vi "Start Batch Process.vi"(8 "error in (no error)":errorcluster, 10 "Files to process":path[](array[path]), 11 "Batch Processor in":refnum<class "Batch Processor.lvclass">) -> (0 "error out":errorcluster, 3 "Batch Processor out":refnum<class "Batch Processor.lvclass">)   [LabVIEW 2016, in "Batch Processor.lvclass"]
uses:
  Batch Processor.lvclass
  C:/Github/LabActor/Worker/Worker.lvclass
  NHMFL_Core/Libraries/Instruments/Instrument Driver/Worker State.ctl
  Worker/Worker.lvclass/Worker.ctl
  NHMFL_Core/Libraries/Instruments/Results/File Path Result/File Path Result.lvclass
  C:/Github/NHMFL_Core/Libraries/Instruments/Results/Acquired Result/Acquired Result.lvclass
  Batch Processor.lvclass/Batch Processor.ctl
  Template Module/Read State.vi
  Template Module/Write State.vi
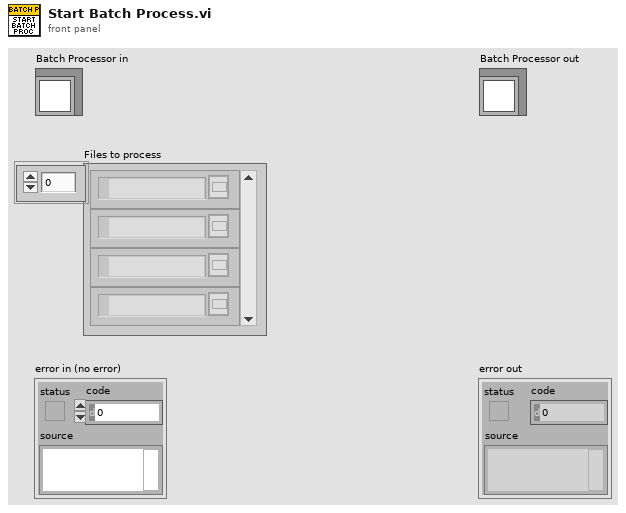
[diagram p1: front panel]
types:
  T1 = typedef "Worker State.ctl" = enum16{"Idle", "Starting", "Working", "Stopping"}
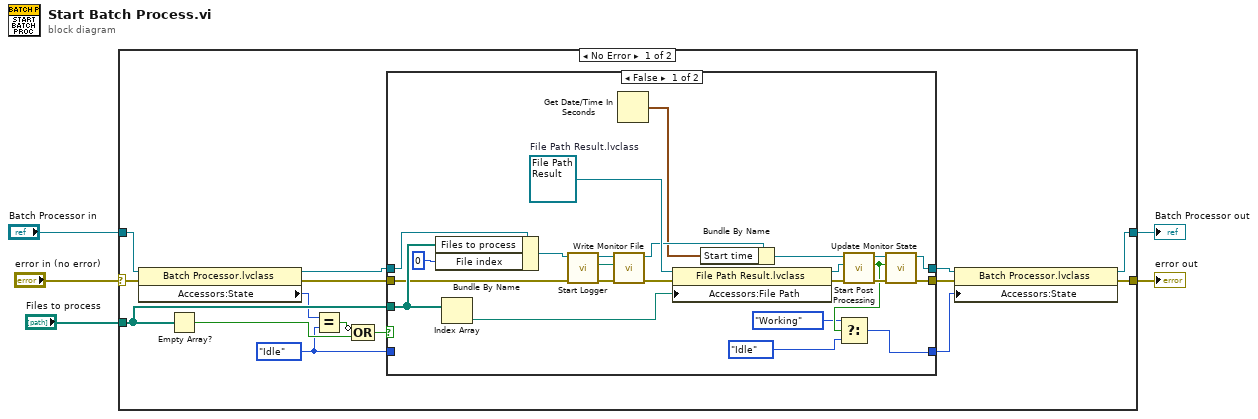
[diagram p0: block diagram]
diagram:
  n1 = case shown="No Error" "error in (no error)" {
    selector: "error in (no error)" -> [w20 w49]
    tunnel: [w6 w49] -> w4
    tunnel: [w7 w48] -> w2
    tunnel: "Batch Processor in" -> [w16 w48]
    tunnel: "Files to process" -> [w19 _]
    frame No Error {
      w9 = Worker_State."Idle" ("State")
      n2 = property class="Batch Processor.lvclass"(reference=w16, error in=w20) -> (reference out=w15:refnum<class "Batch Processor.lvclass">, error out=w17:errorcluster, "Accessors:State"=w12:T1)
      n3 = Empty Array?(array=w19) -> (empty?=w18:bool)
      n4 = Equal?(x=w12, y=w9) -> (x = y?=w13:bool)
      n5 = Compound Arithmetic op=OR(invert w13, w18) -> (w14:bool)
      n6 = case shown="False" w14 {
        tunnel: w15 -> [w44 w46]
        tunnel: w19 -> [w41 _]
        tunnel: w17 -> [w36 w47]
        tunnel: [w29 w46] -> w11
        tunnel: [w28 w47] -> w8
        tunnel: [w23 w45] -> w10
        tunnel: w9 -> [_ w45]
        frame False {
          w42 = refnum<class "File Path Result.lvclass"> refnum  # File Path Result.lvclass
          n7 = Bundle By Name(cluster=w44, "Files to process"=w41, "File index"=0) -> (w37:refnum<class "Batch Processor.lvclass">)
          n8 = Index Array(array=w41) -> (element=w40:path)  [unwired: 1 in]
          n9 = call-dynamic "Start Logger.vi"("error in (no error)"=w36, "Measure Controller in"=w37) -> ("error out"=w33:errorcluster, "File Path"=w31:path, "Measure Controller out"=w35:refnum<class "Batch Processor.lvclass">)  [unwired: 6 in, 1 out]
          n10 = call-dynamic "Write Monitor File.vi"("error in (no error)"=w33, "Monitor File"=w31, "Monitor-Pulse in"=w35) -> ("error out"=w32:errorcluster, "Monitor-Pulse out"=w34:refnum<class "Batch Processor.lvclass">)  [unwired: 7 in]
          n11 = Get Date/Time In Seconds() -> (seconds since 1Jan1904=w25:timestamp)
          n12 = property class="File Path Result.lvclass"(reference=w42, error in=w32, "Accessors:File Path"=w40) -> (reference out=w39:refnum<class "File Path Result.lvclass">, error out=w38:errorcluster)
          n13 = Bundle By Name(cluster=w34, "Start time"=w25) -> (w26:refnum<class "Batch Processor.lvclass">)
          n14 = call-dynamic "Start Post Processing.vi"("error in (no error)"=w38, "Result in"=w39, "Monitor-Pulse in"=w26) -> ("error out"=w27:errorcluster, "Started"=w24:bool, "Monitor-Pulse out"=w30:refnum<class "Batch Processor.lvclass">)  [unwired: 6 in]
          n15 = Select(t=Worker_State."Working", s=w24, f=Worker_State."Idle" ("State")) -> (s? t:f=w23:T1)
          n16 = call-dynamic "Update Monitor State.vi"("error in (no error)"=w27, "Monitor Running"=w24, "Monitor-Pulse in"=w30) -> ("error out"=w28:errorcluster, "Monitor-Pulse out"=w29:refnum<class "Batch Processor.lvclass">)  [unwired: 7 in]
        }
        frame True {
        }
      }
      n17 = property class="Batch Processor.lvclass"(reference=w11, error in=w8, "Accessors:State"=w10) -> (reference out=w7:refnum<class "Batch Processor.lvclass">, error out=w6:errorcluster)
    }
    frame Error {
    }
  }
  "error out" <- w4
  "Batch Processor out" <- w2
